vi "test-Function-Generator-ALL-TESTS.vi"(8 "error in (no error)":errorcluster) -> (0 "error out":errorcluster, 3 "All Passed":bool)   [LabVIEW 2019]
panel:
  out "Test 3":bool
  out "Test 1":bool
  out "Test 2":bool
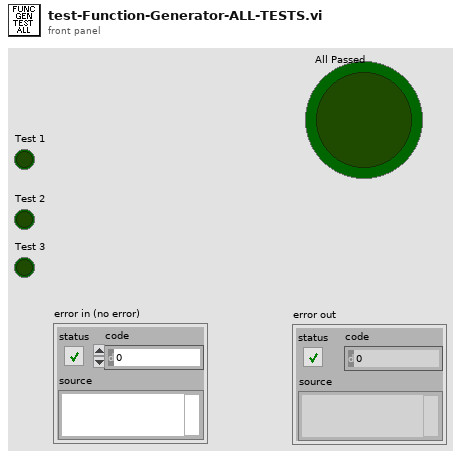
[diagram p1: front panel]
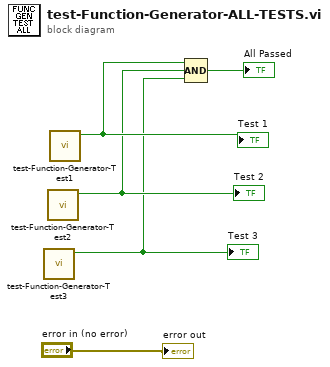
[diagram p0: block diagram]
diagram:
  n1 = call "test-Function-Generator-Test3.vi"() -> ("All tests passed"=w1:bool)  [unwired: 10 in, 1 out]
  "Test 3" <- w1
  n2 = call "test-Function-Generator-Test2.vi"() -> ("All tests passed"=w2:bool)  [unwired: 10 in, 1 out]
  "Test 2" <- w2
  n3 = call "test-Function-Generator-Test1.vi"() -> ("All tests passed"=w3:bool)  [unwired: 10 in, 1 out]
  "Test 1" <- w3
  n4 = Compound Arithmetic op=AND(w3, w2, w1) -> (→"All Passed":bool)
  "error out" <- "error in (no error)"
